vi "Destroy.vi"(8 "ErrorIn":errorcluster, 11 "ReferenceIn":refnum<class "AppConfigJSON.lvclass">) -> (0 "ErrorOut":errorcluster, 3 "ReferenceOut":refnum<class "AppConfigJSON.lvclass">)   [LabVIEW 2021, in "AppConfigJSON.lvclass"]
uses:
  AppConfigJSON.lvclass
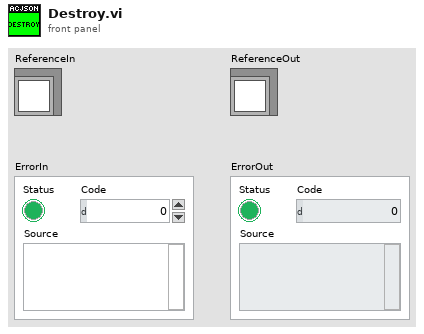
[diagram p1: front panel]
types:
  T1 = typedef "AppConfigJSON.lvclass/ObjectAttributes.ctl" = cluster{"Name":string, "ConfigFilePath":path, "Objects":T2[], "ApplicationBasePath":path, "ObjectName":string}
  T2 = typedef "IApplicationConfiguration.lvclass/ObjectDataDetails.ctl" = cluster{"ObjectName":string, "ObjectType":string, "Interfaces":T3[]}
  T3 = typedef "IApplicationConfiguration.lvclass/ObjectData.ctl" = cluster{"Label":string, "ObjectName":string, "Type":string}
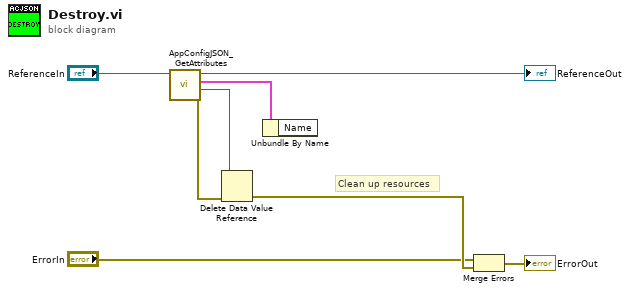
[diagram p0: block diagram]
diagram:
  # "Clean up resources"
  n1 = call "AppConfigJSON_GetAttributes.vi"("ReferenceIn"="ReferenceIn") -> ("ErrorOut"=w7:errorcluster, "DataRef"=w2:refnum<data-value>, "Data"=w1:T1, "ReferenceOut"=→"ReferenceOut":refnum<class "AppConfigJSON.lvclass">)  [unwired: 7 in]
  n2 = Delete Data Value Reference(data value reference=w2, error in=w7) -> (error out=w6:errorcluster)  [unwired: 1 out]
  n3 = Unbundle By Name(w1) -> ()  [unwired: 1 out]
  n4 = Merge Errors("ErrorIn", w6) -> (→"ErrorOut":errorcluster)
